vi "Sim drop out (SubVI).vi"(11 "Drop-Out Out in":i16[](array[numeric])) -> (3 "Drop-Out Out out":i16[](array[numeric]))   [LabVIEW 2014, in "Vessel.lvclass"]
uses:
  ROV/Vessel.lvclass
panel:
  in  "Sim Drop-Out Out":i16[](array[numeric])
  in  "drop out":bool
  # "North"
  # "East"
  # "Depth"
  # "Roll"
  # "Pitch"
  # "Yaw"
  # "Surge"
  # "Sway"
  # "Heave"
  # "p"
  # "q"
  # "r"
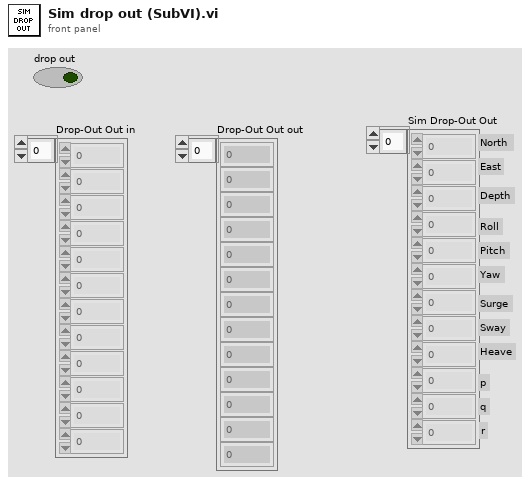
[diagram p1: front panel]
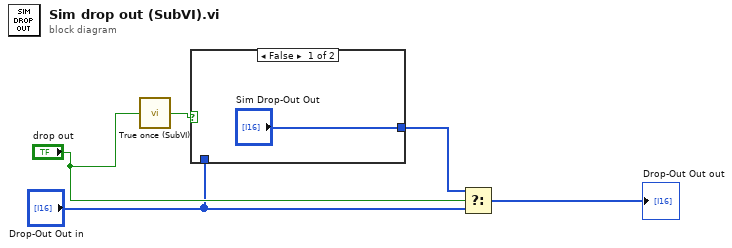
[diagram p0: block diagram]
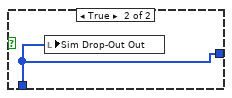
[diagram p2: hidden frame]
diagram:
  n1 = call "True once (SubVI).vi"("Automatic"="drop out") -> ("Boolean"=w3:bool)
  n2 = case shown="False" w3 {
    tunnel: "Drop-Out Out in" -> [_ w7]
    tunnel: ["Sim Drop-Out Out" w7] -> w1
    frame False {
    }
    frame True {
      n3 = local write "Sim Drop-Out Out"(w7) -> ()
    }
  }
  n4 = Select(t=w1, s="drop out", f="Drop-Out Out in") -> (s? t:f=→"Drop-Out Out out":i16[])
